vi "RemoteDCPowerSession_CallInitializeMeasurementLinkSessionWithAttachBehavior_RemoteSessionAttached.vi"(8 "error in (no error)":errorcluster) -> (0 "error out":errorcluster, 2 "result":string, 3 "pass":bool)   [LabVIEW 2020, in "MeasurementServerTests.lvlib"]
uses:
  MeasurementServerTests.lvlib
  Runtime/MeasurementLink niDCPower/Instrument/Instrument.lvclass
  Runtime/MeasurementLink Instrument/IInstrument/Initialize Session Behavior.ctl
  Runtime/MeasurementLink Instrument/IInstrument/IInstrument.lvclass
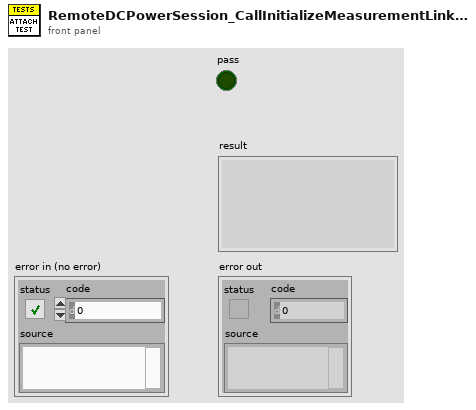
[diagram p1: front panel]
types:
  T1 = typedef "MeasurementLink Instrument.lvlib/IInstrument.lvclass/Remote Connection Options.ctl" = cluster{"session name":string, "address":string, "port":u32}
  T2 = typedef "MeasurementLink Instrument.lvlib/IInstrument.lvclass/Initialize Session Behavior.ctl" = enum16{"Create Session", "Attach Session"}
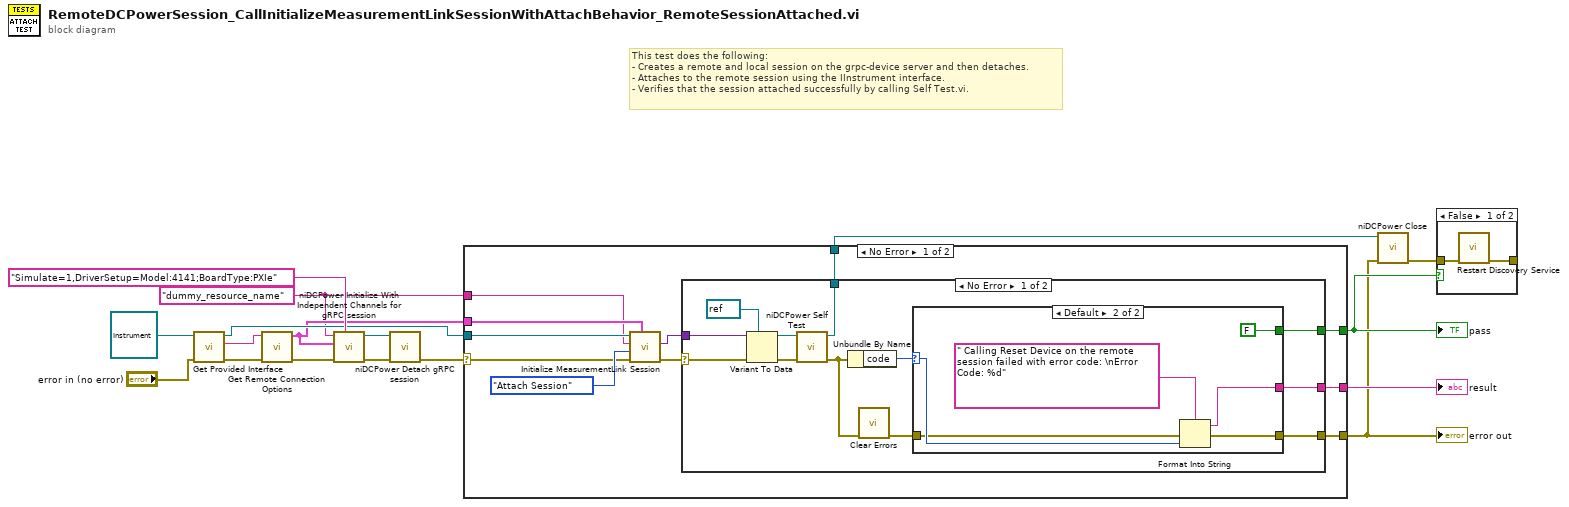
[diagram p0: block diagram]
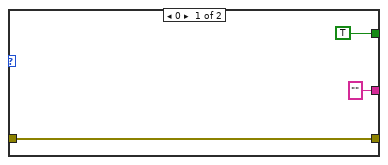
[diagram p2: hidden frame]
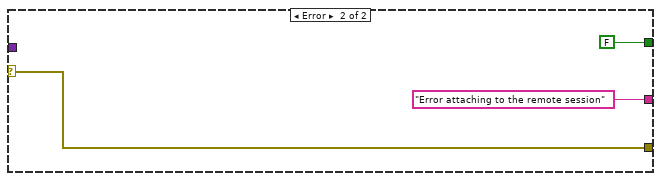
[diagram p3: hidden frame]
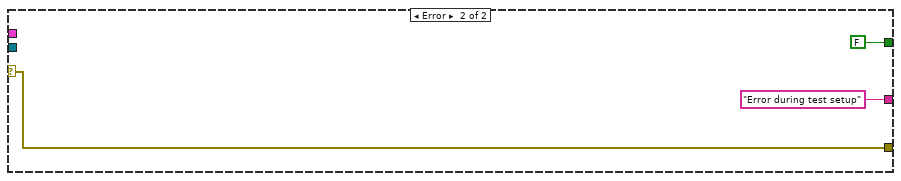
[diagram p4: hidden frame]
diagram:
  w1 = "dummy_resource_name" ("resource name")
  # "This test does the following:\n- Creates a remote and local session on the grpc-device server and then detaches.\n- Attaches to the remote session using the IInstrument interface.\n- Verifies that the session attached successfully by calling Self Test.vi."
  n1 = call-dynamic "Get Provided Interface.vi"("error in (no error)"="error in (no error)", "instrument in"=refnum<class "Instrument.lvclass"> refnum ("MeasurementLink niDCPower.lvlib:Instrument.lvclass")) -> ("error out"=w9:errorcluster, "provided interface"=w8:string, "instrument out"=w6:refnum<class "Instrument.lvclass">)  [unwired: 7 in]
  n2 = call "Get Remote Connection Options.vi"("error in (no error)"=w9, "provided interface"=w8) -> ("error out"=w11:errorcluster, "remote connection options"=w2:T1)  [unwired: 8 in]
  n3 = call <instrlib>:"niDCPower Initialize With Independent Channels for gRPC session.vi"("option string"="Simulate=1,DriverSetup=Model:4141;BoardType:PXIe", "error in (no error)"=w11, "gRPC options"=w2, "resource name"=w1) -> ("error out"=w5:errorcluster, "instrument handle out"=w3:refnum<k15>)  [unwired: 6 in]
  n4 = call <instrlib>:"niDCPower Detach gRPC session.vi"("error in (no error)"=w5, "instrument handle"=w3) -> ("error out"=w4:errorcluster)  [unwired: 9 in]
  n5 = case shown="No Error" w4 {
    selector: w4 -> [w22 w53]
    tunnel: [w27 w53] -> w13
    tunnel: [w28 FALSE] -> w14
    tunnel: [w26 "Error during test setup" ("f")] -> w17
    tunnel: w6 -> [w21 _]
    tunnel: [w20 _] -> w16
    tunnel: w2 -> [w19 _]
    tunnel: w1 -> [w18 _]
    frame No Error {
      n6 = call-dynamic "Initialize MeasurementLink Session.vi"("remote connection options"=w19, "error in (no error)"=w22, "initialize session behavior"=Initialize_Session_Behavior."Attach Session", "resource name"=w18, "instrument in"=w21) -> ("error out"=w24:errorcluster, "session out"=w25:variant)  [unwired: 4 in, 1 out]
      n7 = case shown="No Error" w24 {
        selector: w24 -> [w34 w51]
        tunnel: [w40 FALSE] -> w28
        tunnel: [w30 w51] -> w27
        tunnel: [w37 "Error attaching to the remote session"] -> w26
        tunnel: w25 -> [w35 _]
        tunnel: [w29 _] -> w20
        frame No Error {
          n8 = Variant To Data(error in=w34, type=refnum<k15> refnum ("instrument handle"), Variant=w35) -> (data=w31:refnum<k15>, error out=w32:errorcluster)
          n9 = call <instrlib>:"niDCPower Self Test.vi"("error in (no error)"=w32, "instrument handle"=w31) -> ("error out"=w36:errorcluster, "instrument handle out"=w29:refnum<k15>)  [unwired: 6 in, 2 out]
          n10 = Unbundle By Name(w36) -> ("code"=w39:i32)
          n11 = call <vilib>:"Clear Errors.vi"("error in (no error)"=w36) -> ("error out"=w38:errorcluster)  [unwired: 5 in, 1 out]
          n12 = case shown="Default" w39 {
            selector: w39 -> [_ w48]
            tunnel: ["" w47] -> w37
            tunnel: [TRUE FALSE] -> w40
            tunnel: w38 -> [w42 w45]
            tunnel: [w42 w44] -> w30
            frame 0 {
            }
            frame Default {
              n13 = Format Into String(format string=" Calling Reset Device on the remote session failed with error code: \nError Code: %d" ("f"), error in=w45, w48) -> (resulting string=w47:string, error out=w44:errorcluster)  [unwired: 1 in]
            }
          }
        }
        frame Error {
        }
      }
    }
    frame Error {
    }
  }
  "error out" <- w13
  "pass" <- w14
  "result" <- w17
  n14 = call <instrlib>:"niDCPower Close.vi"("error in (no error)"=w13, "instrument handle"=w16) -> ("error out"=w15:errorcluster)  [unwired: 9 in]
  n15 = case shown="False" w14 {
    tunnel: w15 -> [w57 _]
    tunnel: [w56 _] -> _
    frame False {
      n16 = call "Restart Discovery Service.vi"("error in"=w57) -> ("error out"=w56:errorcluster)  [unwired: 10 in]
    }
    frame True {
    }
  }
